vi "Auto Scale.vi"(11 "Right?":bool=TRUE) -> ()   [LabVIEW 2017]
uses:
  Auto Scale Type Def.ctl
  LabVIEW_is_Under_Control.lib/Util/Unpack Gamepad/D-Pad.ctl
  LabVIEW_is_Under_Control.lib/Util/Unpack Gamepad/Button Cluster.ctl
  Team Code/Robot Global Data.vi
panel:
  in  "Time_Limit_fwd 3":dbl=1000.0 format="%#_13g"
  in  "Delay Fwd 3":i32=100
  in  "DistanceFwd 3":dbl=-60.0
  in  "Time to wait 3 (min 50ms)":dbl=100.0
  in  "Time_Limit_fwd 2":dbl=1000.0 format="%#_13g"
  in  "Delay Fwd 2":i32=100
  in  "DistanceFwd 2":dbl=55.0
  in  "Time to wait 2 (min 50ms)":dbl=100.0
  out "Auto state":T1=enum."Finalizando"
  in  "Delay Turn":i32=100
  in  "Turn":dbl=-30.0 format="%#_13g"
  in  "Time_Limit_Turn":dbl=1000.0 format="%#_13g"
  in  "Time_Limit_fwd":dbl=5000.0 format="%#_13g"
  in  "Delay Fwd":i32=300
  in  "DistanceFwd":dbl=600.0
  in  "Time to wait (min 50ms)":dbl=100.0
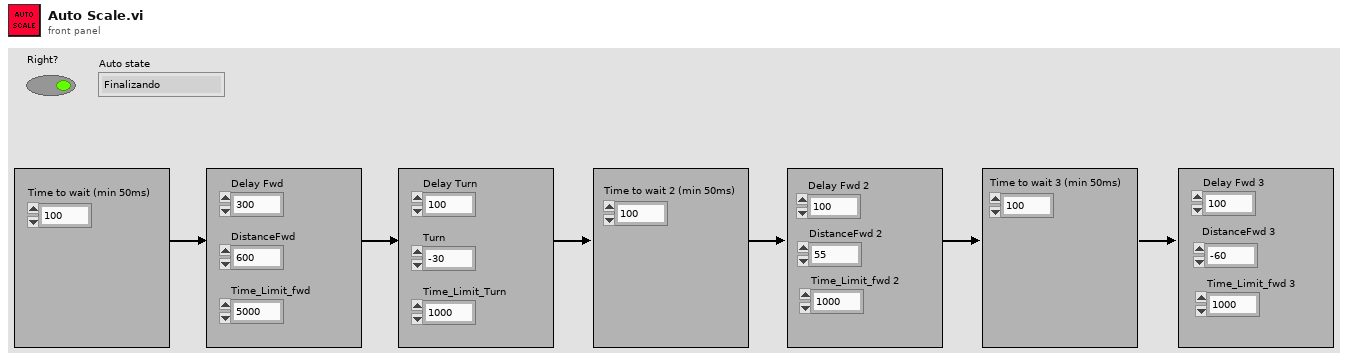
[diagram p1: front panel]
types:
  T1 = typedef "Auto Scale Type Def.ctl" = enum16{"Zerandosensor", "Andando", "Girando", "Zerandosensor2", "Andando2", "Score", "Zerandosensor3", "Andando3", "Finalizando"}
  T2 = typedef "D-Pad.ctl" = cluster{"Top":bool, "Bottom":bool, "None":bool, "Right":bool, "Left":bool}
  T3 = cluster{"proportional gain (Kc)":dbl, "integral time (Ti, min)":dbl, "derivative time (Td, min)":dbl}
  T4 = typedef "Button Cluster.ctl" = cluster{"Buttons[0]":bool, "Buttons[1]":bool, "Buttons[2]":bool, "Buttons[3]":bool, "Buttons[4]":bool, "Buttons[5]":bool, "Buttons[6]":bool, "Buttons[7]":bool, "Buttons[8]":bool, "Buttons[9]":bool}
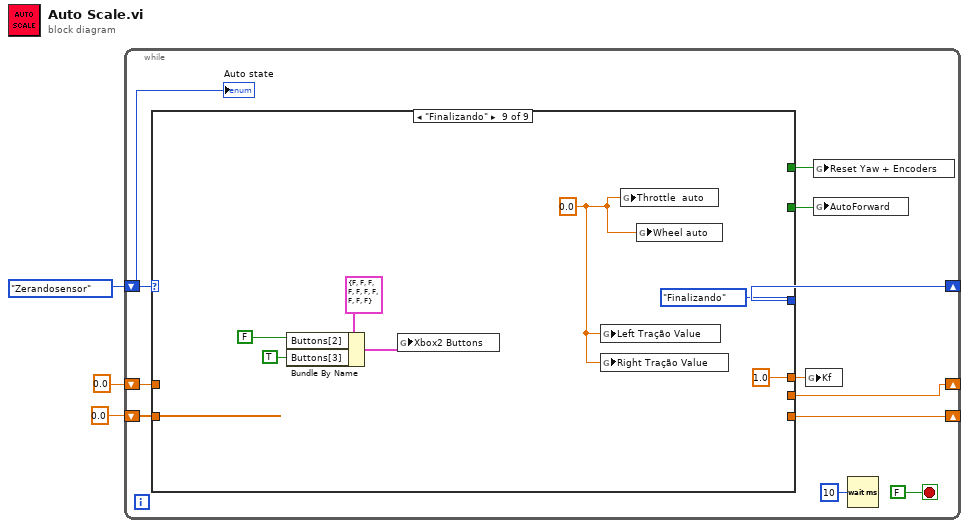
[diagram p0: block diagram]
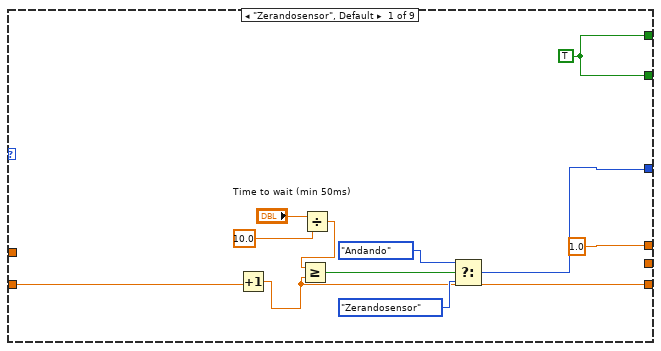
[diagram p2: hidden frame]
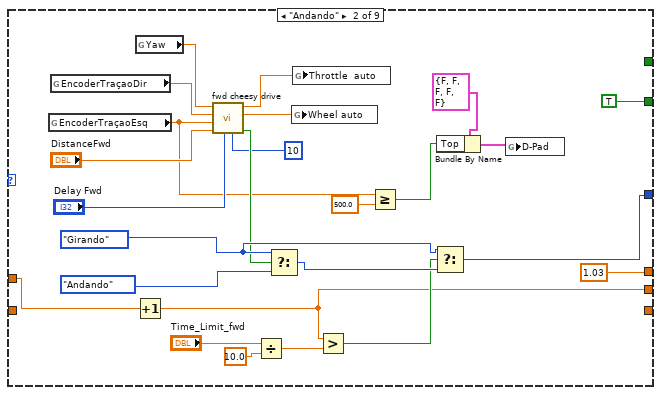
[diagram p3: hidden frame]
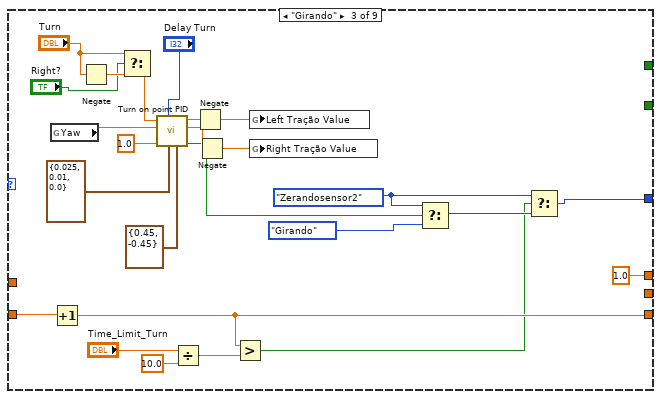
[diagram p4: hidden frame]
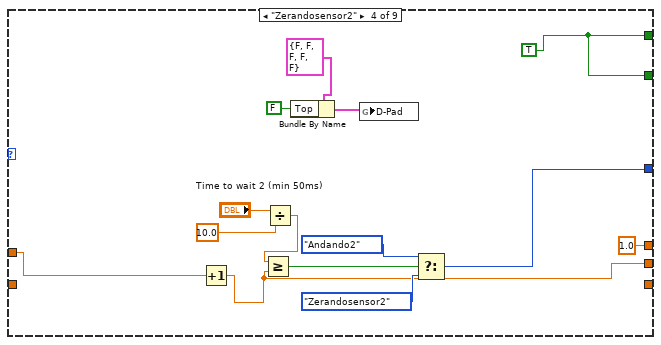
[diagram p5: hidden frame]
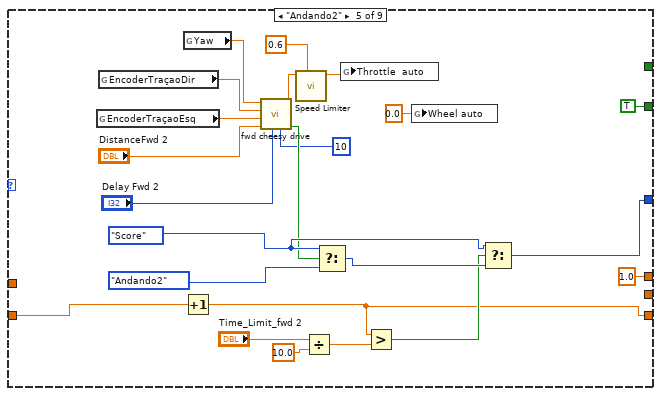
[diagram p6: hidden frame]
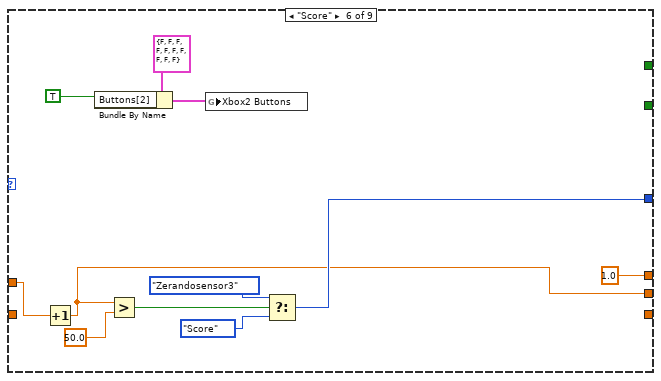
[diagram p7: hidden frame]
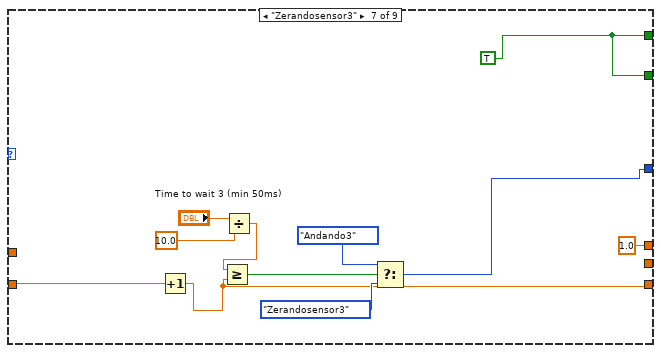
[diagram p8: hidden frame]
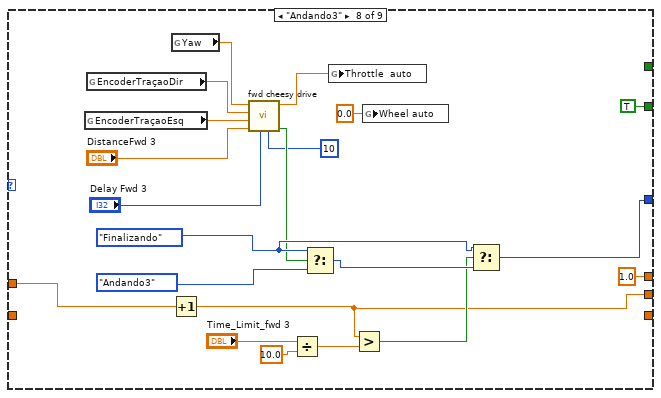
[diagram p9: hidden frame]
diagram:
  n1 = while {
    shift-right: [w9] -> _
    shift-left: Auto_Scale_Type_Def."Zerandosensor" -> [w12]
    shift-right: [w10] -> _
    shift-left: 0.0 -> [w11]
    shift-right: [w4] -> _
    shift-left: 0.0 -> [w5]
    stop <- FALSE stop-if-true
    n2 = case shown="\"Finalizando\"" w12 {
      tunnel: w11 -> [w21 _ w71 _ w98 _ w126 _ _]
      tunnel: [w18 _ w70 _ w97 _ w125 _ _] -> w10
      tunnel: [w17 w43 w55 w80 w95 w115 w127 w137 Auto_Scale_Type_Def."Finalizando"] -> w9
      tunnel: [w16 _ _ w79 _ _ w128 _ _] -> w7
      tunnel: [w16 TRUE _ w79 TRUE _ w128 TRUE _] -> w6
      tunnel: [1.0 1.03 1.0 1.0 1.0 1.0 1.0 1.0 1.0] -> w8
      tunnel: w5 -> [_ w33 _ w83 _ w114 _ w140 _]
      tunnel: [_ w32 _ w82 _ w113 _ w139 _] -> w4
      frame "Zerandosensor", Default {
        w16 = TRUE
        n3 = Increment(x=w21) -> (x+1=w18:dbl)
        n4 = Divide(x="Time to wait (min 50ms)", y=10.0) -> (x/y=w23:dbl)
        n5 = Greater Or Equal?(x=w23, y=w18) -> (x >= y?=w22:bool)
        n6 = Select(t=Auto_Scale_Type_Def."Andando", s=w22, f=Auto_Scale_Type_Def."Zerandosensor") -> (s? t:f=w17:T1)
      }
      frame "Andando" {
        w36 = Auto_Scale_Type_Def."Girando"
        n7 = global read "Robot Global Data.vi" "EncoderTraçaoEsq"() -> (w27:dbl)
        n8 = global read "Robot Global Data.vi" "EncoderTraçaoDir"() -> (w49:dbl)
        n9 = Increment(x=w33) -> (x+1=w32:dbl)
        n10 = global read "Robot Global Data.vi" "Yaw"() -> (w50:dbl)
        n11 = call "fwd cheesy drive.vi"("Loop Timer"=10, "Time to stop"="Delay Fwd", "Distance"="DistanceFwd", "Encoder Left"=w27, "Encoder Right"=w49, "Yaw"=w50) -> ("Finished distance"=w34:bool, "Direction"=w47:dbl, "Trottle"=w46:dbl)  [unwired: 2 in, 1 out]
        n12 = Divide(x="Time_Limit_fwd", y=10.0) -> (x/y=w41:dbl)
        n13 = Select(t=w36, s=w34, f=Auto_Scale_Type_Def."Andando") -> (s? t:f=w44:T1)
        n14 = global write "Robot Global Data.vi" "Wheel auto"(w47) -> ()
        n15 = global write "Robot Global Data.vi" "Throttle  auto"(w46) -> ()
        n16 = Greater?(x=w32, y=w41) -> (0:w38:bool)
        n17 = Greater Or Equal?(x=w27, y=500.0) -> (x >= y?=w28:bool)
        n18 = Select(t=w36, s=w38, f=w44) -> (s? t:f=w43:T1)
        n19 = Bundle By Name(cluster=T2 {"Top"=FALSE, "Bottom"=FALSE, "None"=FALSE, "Right"=FALSE, "Left"=FALSE} ("D-Pad"), "Top"=w28) -> (w30:T2)
        n20 = global write "Robot Global Data.vi" "D-Pad"(w30) -> ()
      }
      frame "Girando" {
        w57 = Auto_Scale_Type_Def."Zerandosensor2"
        n21 = global read "Robot Global Data.vi" "Yaw"() -> (w66:dbl)
        n22 = Increment(x=w71) -> (x+1=w70:dbl)
        n23 = Negate(x="Turn") -> (-x=w54:dbl)
        n24 = Select(t="Turn", s="Right?", f=w54) -> (s? t:f=w51:dbl)
        n25 = call "Turn on point PID.vi"("Range"=cluster{"output high":dbl, "output low":dbl} {"output high"=0.45, "output low"=-0.45}, "Gains"=T3 {"proportional gain (Kc)"=0.025, "integral time (Ti, min)"=0.01, "derivative time (Td, min)"=0.0}, "Time to stop"="Delay Turn", "Precision"=1.0, "Yaw"=w66, "Setpoint(degrees)"=w51) -> ("Finished?"=w62:bool, "PWM right"=w65:dbl, "PWM left"=w64:dbl)  [unwired: 3 in]
        n26 = Divide(x="Time_Limit_Turn", y=10.0) -> (x/y=w73:dbl)
        n27 = Negate(x=w64) -> (-x=w67:dbl)
        n28 = Negate(x=w65) -> (-x=w68:dbl)
        n29 = Greater?(x=w70, y=w73) -> (0:w58:bool)
        n30 = global write "Robot Global Data.vi" "Left Tração Value"(w67) -> ()
        n31 = global write "Robot Global Data.vi" "Right Tração Value"(w68) -> ()
        n32 = Select(t=w57, s=w62, f=Auto_Scale_Type_Def."Girando") -> (s? t:f=w69:T1)
        n33 = Select(t=w57, s=w58, f=w69) -> (s? t:f=w55:T1)
      }
      frame "Zerandosensor2" {
        w79 = TRUE
        n34 = Increment(x=w83) -> (x+1=w82:dbl)
        n35 = Divide(x="Time to wait 2 (min 50ms)", y=10.0) -> (x/y=w87:dbl)
        n36 = Greater Or Equal?(x=w87, y=w82) -> (x >= y?=w86:bool)
        n37 = Bundle By Name(cluster=T2 {"Top"=FALSE, "Bottom"=FALSE, "None"=FALSE, "Right"=FALSE, "Left"=FALSE} ("D-Pad"), "Top"=FALSE) -> (w78:T2)
        n38 = global write "Robot Global Data.vi" "D-Pad"(w78) -> ()
        n39 = Select(t=Auto_Scale_Type_Def."Andando2", s=w86, f=Auto_Scale_Type_Def."Zerandosensor2") -> (s? t:f=w80:T1)
      }
      frame "Andando2" {
        w102 = Auto_Scale_Type_Def."Score"
        n40 = global read "Robot Global Data.vi" "EncoderTraçaoEsq"() -> (w111:dbl)
        n41 = global read "Robot Global Data.vi" "EncoderTraçaoDir"() -> (w110:dbl)
        n42 = Increment(x=w98) -> (x+1=w97:dbl)
        n43 = global read "Robot Global Data.vi" "Yaw"() -> (w112:dbl)
        n44 = call "fwd cheesy drive.vi"("Loop Timer"=10, "Time to stop"="Delay Fwd 2", "Distance"="DistanceFwd 2", "Encoder Left"=w111, "Encoder Right"=w110, "Yaw"=w112) -> ("Finished distance"=w100:bool, "Trottle"=w91:dbl)  [unwired: 2 in, 2 out]
        n45 = call "Speed Limiter.vi"("Limit"=0.6, "Motor Input"=w91) -> ("Output"=w92:dbl)  [unwired: 9 in]
        n46 = Divide(x="Time_Limit_fwd 2", y=10.0) -> (x/y=w106:dbl)
        n47 = Select(t=w102, s=w100, f=Auto_Scale_Type_Def."Andando2") -> (s? t:f=w107:T1)
        n48 = global write "Robot Global Data.vi" "Throttle  auto"(w92) -> ()
        n49 = Greater?(x=w97, y=w106) -> (0:w103:bool)
        n50 = global write "Robot Global Data.vi" "Wheel auto"(0.0 ("Wheel auto")) -> ()
        n51 = Select(t=w102, s=w103, f=w107) -> (s? t:f=w95:T1)
      }
      frame "Score" {
        n52 = Increment(x=w114) -> (x+1=w113:dbl)
        n53 = Bundle By Name(cluster=T4 {"Buttons[0]"=FALSE, "Buttons[1]"=FALSE, "Buttons[2]"=FALSE, "Buttons[3]"=FALSE, "Buttons[4]"=FALSE, "Buttons[5]"=FALSE, "Buttons[6]"=FALSE, "Buttons[7]"=FALSE, "Buttons[8]"=FALSE, "Buttons[9]"=FALSE} ("Xbox Buttons"), "Buttons[2]"=TRUE) -> (w122:T4)
        n54 = Greater?(x=w113, y=50.0) -> (0:w118:bool)
        n55 = global write "Robot Global Data.vi" "Xbox2 Buttons"(w122) -> ()
        n56 = Select(t=Auto_Scale_Type_Def."Zerandosensor3", s=w118, f=Auto_Scale_Type_Def."Score") -> (s? t:f=w115:T1)
      }
      frame "Zerandosensor3" {
        w128 = TRUE
        n57 = Increment(x=w126) -> (x+1=w125:dbl)
        n58 = Divide(x="Time to wait 3 (min 50ms)", y=10.0) -> (x/y=w132:dbl)
        n59 = Greater Or Equal?(x=w132, y=w125) -> (x >= y?=w131:bool)
        n60 = Select(t=Auto_Scale_Type_Def."Andando3", s=w131, f=Auto_Scale_Type_Def."Zerandosensor3") -> (s? t:f=w127:T1)
      }
      frame "Andando3" {
        w144 = Auto_Scale_Type_Def."Finalizando"
        n61 = global read "Robot Global Data.vi" "EncoderTraçaoEsq"() -> (w154:dbl)
        n62 = global read "Robot Global Data.vi" "EncoderTraçaoDir"() -> (w153:dbl)
        n63 = Increment(x=w140) -> (x+1=w139:dbl)
        n64 = global read "Robot Global Data.vi" "Yaw"() -> (w155:dbl)
        n65 = call "fwd cheesy drive.vi"("Loop Timer"=10, "Time to stop"="Delay Fwd 3", "Distance"="DistanceFwd 3", "Encoder Left"=w154, "Encoder Right"=w153, "Yaw"=w155) -> ("Finished distance"=w142:bool, "Trottle"=w151:dbl)  [unwired: 2 in, 2 out]
        n66 = Divide(x="Time_Limit_fwd 3", y=10.0) -> (x/y=w148:dbl)
        n67 = Select(t=w144, s=w142, f=Auto_Scale_Type_Def."Andando3") -> (s? t:f=w149:T1)
        n68 = global write "Robot Global Data.vi" "Throttle  auto"(w151) -> ()
        n69 = Greater?(x=w139, y=w148) -> (0:w145:bool)
        n70 = global write "Robot Global Data.vi" "Wheel auto"(0.0 ("Wheel auto")) -> ()
        n71 = Select(t=w144, s=w145, f=w149) -> (s? t:f=w137:T1)
      }
      frame "Finalizando" {
        w156 = 0.0
        n72 = Bundle By Name(cluster=T4 {"Buttons[0]"=FALSE, "Buttons[1]"=FALSE, "Buttons[2]"=FALSE, "Buttons[3]"=FALSE, "Buttons[4]"=FALSE, "Buttons[5]"=FALSE, "Buttons[6]"=FALSE, "Buttons[7]"=FALSE, "Buttons[8]"=FALSE, "Buttons[9]"=FALSE} ("Xbox Buttons"), "Buttons[2]"=FALSE, "Buttons[3]"=TRUE) -> (w158:T4)
        n73 = global write "Robot Global Data.vi" "Xbox2 Buttons"(w158) -> ()
        n74 = global write "Robot Global Data.vi" "Left Tração Value"(w156) -> ()
        n75 = global write "Robot Global Data.vi" "Right Tração Value"(w156) -> ()
        n76 = global write "Robot Global Data.vi" "Throttle  auto"(w156) -> ()
        n77 = global write "Robot Global Data.vi" "Wheel auto"(w156) -> ()
      }
    }
    n78 = global write "Robot Global Data.vi" "Kf"(w8) -> ()
    n79 = global write "Robot Global Data.vi" "Reset Yaw + Encoders"(w7) -> ()
    n80 = global write "Robot Global Data.vi" "AutoForward"(w6) -> ()
    n81 = Wait (ms)(milliseconds to wait=u32 10) -> ()  [unwired: 1 out]
    "Auto state" <- w12
  }
